vi "UpdateDB_PV3.vi"(3 "value precision (0.01)":dbl=0.01, 4 "trace name":string, 5 "process name":string, 6 "error in (no error)":errorcluster, 7 "Time Stamp":timestamp, 8 "Double":dbl, 9 "database URL":path) -> (0 "error out":errorcluster)   [LabVIEW 2013]
uses:
  <vilib>/lvdsc/historical/Open Trace (Numeric).vi
  <vilib>/lvdsc/historical/Write Trace (Numeric).vi
  <vilib>/lvdsc/NI_DSC.lvlib
panel:
  out "database URL out":path
  out "x-y":dbl
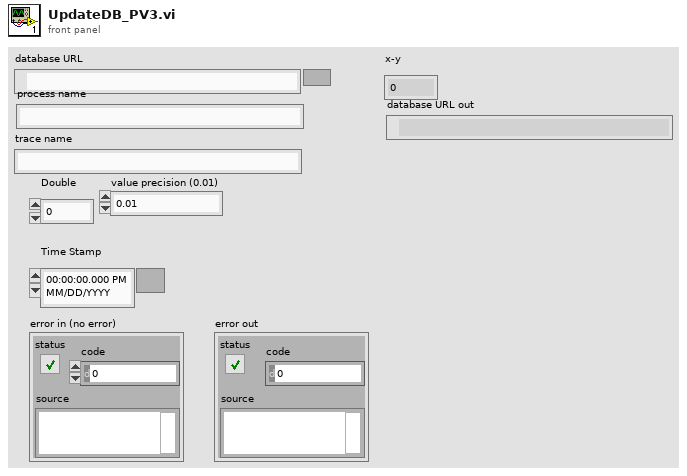
[diagram p1: front panel]
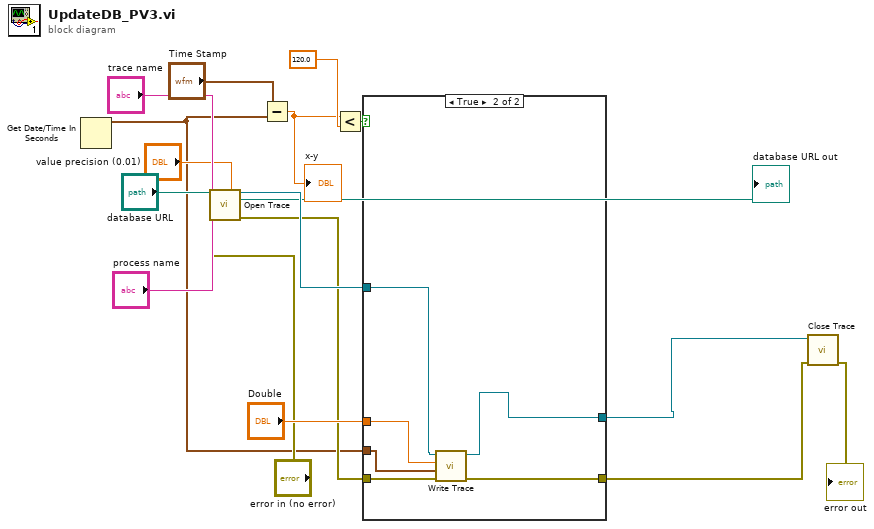
[diagram p0: block diagram]
diagram:
  n1 = Get Date/Time In Seconds() -> (seconds since 1Jan1904=w1:timestamp)
  n2 = call-poly <vilib>:"Open Trace.vi"("database URL"="database URL", "value precision (0.01)"="value precision (0.01)", "process name"="process name", "trace name"="trace name", "error in (no error)"="error in (no error)") -> ("trace reference"=w13:refnum<k1>, "database URL out"=→"database URL out":path, "error out"=w6:errorcluster)  [unwired: 8 in]
  n3 = Subtract(x="Time Stamp", y=w1) -> (x-y=w14:dbl)
  "x-y" <- w14
  n4 = Less?(x=w14, y=120.0 ("x")) -> (x < y?=w17:bool)
  n5 = case shown="True" w17 {
    tunnel: w6 -> [w19 w25]
    tunnel: [w19 w24] -> w4
    tunnel: "Double" -> [_ w23]
    tunnel: w1 -> [_ w22]
    tunnel: w13 -> [w18 w21]
    tunnel: [w18 w20] -> w8
    frame False {
    }
    frame True {
      n6 = call-poly <vilib>:"Write Trace.vi"("error in (no error)"=w25, "timestamp (now)"=w22, "value"=w23, "trace ref"=w21) -> ("error out"=w24:errorcluster, "trace ref out"=w20:refnum<k1>)  [unwired: 6 in]
    }
  }
  n7 = call <vilib>:"Close Trace.vi"("error in (no error)"=w4, "trace reference"=w8) -> ("error out"=→"error out":errorcluster)  [unwired: 9 in]
